vi "Update Form.vi"(7 "Name":string, 8 "error in (no error)":errorcluster, 10 "Table":refnum<class "Basic Table.lvclass">, 11 "Form Server Wrapper in":refnum<class "Form Server Wrapper.lvclass">) -> (0 "error out":errorcluster, 3 "Form Server Wrapper out":refnum<class "Form Server Wrapper.lvclass">)   [LabVIEW 2020, in "Form Server.lvlib" / "Form Server Wrapper.lvclass"]
uses:
  Form Server Wrapper.lvclass
  Database OOP/Table Libraries/Basic Table/Basic Table Class/Basic Table.lvclass
  Form Server Wrapper.lvclass/Form Server Wrapper.ctl
  Form Server Messages Messages/Update Form Msg/Update Form Msg.lvclass/Update Form Msg.ctl
  <vilib>/ActorFramework/Message Enqueuer/Message Enqueuer.lvclass/Message Enqueuer.ctl
  <vilib>/ActorFramework/Message Enqueuer/Enqueue.vi
  Form Server Messages Messages/Update Form Msg/Update Form Msg.lvclass
  C:/Program Files (x86)/National Instruments/LabVIEW 2020/vi.lib/ActorFramework/Message/Message.lvclass
  <vilib>/ActorFramework/Message Priority Queue/Priority Enqueue.vi
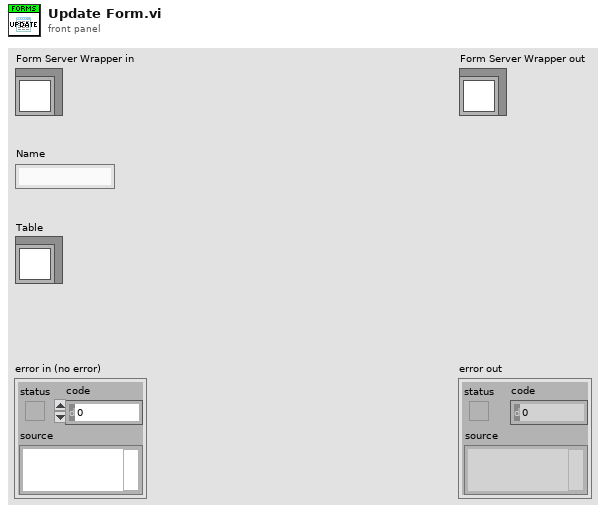
[diagram p1: front panel]
types:
  T1 = typedef "Form Server Interfaces.lvlib/Form ID.ctl" = cluster{"Name":string, "Panel type":string}
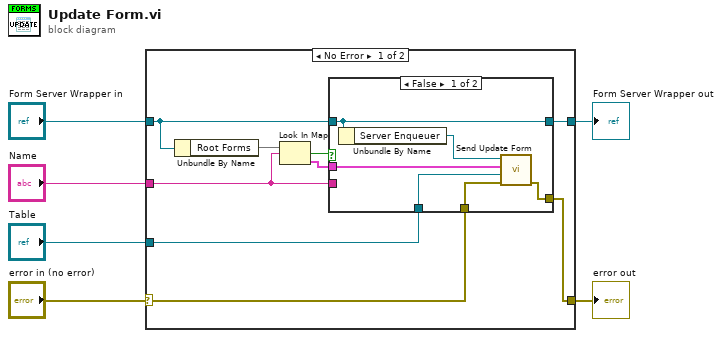
[diagram p0: block diagram]
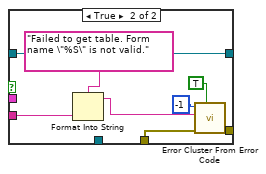
[diagram p2: hidden frame]
diagram:
  n1 = case shown="No Error" "error in (no error)" {
    selector: "error in (no error)" -> [w14 w31]
    tunnel: [w13 w31] -> w4
    tunnel: [w15 w30] -> w5
    tunnel: "Form Server Wrapper in" -> [w12 w30]
    tunnel: "Name" -> [w8 _]
    tunnel: "Table" -> [w7 _]
    frame No Error {
      n2 = Unbundle By Name(w12) -> ("Root Forms"=w11:map{string, T1})
      n3 = Look In Map(map=w11, key=w8) -> (key not found?=w10:bool, value=w9:T1)  [unwired: 1 in]
      n4 = case shown="False" w10 {
        tunnel: w9 -> [w19 _]
        tunnel: w12 -> [w21 w26]
        tunnel: [w21 w26] -> w15
        tunnel: w14 -> [w18 w29]
        tunnel: w8 -> [_ w24]
        tunnel: [w17 w22] -> w13
        tunnel: w7 -> [w16 _]
        frame False {
          n5 = Unbundle By Name(w21) -> ("Server Enqueuer"=w20:refnum<class "Message Enqueuer.lvclass">)
          n6 = call "Send Update Form.vi"("error in (no error)"=w18, "Table"=w16, "Form ID"=w19, "Message Enqueuer"=w20) -> ("error out"=w17:errorcluster)  [unwired: 6 in, 1 out]
        }
        frame True {
          n7 = Format Into String(format string="Failed to get table. Form name \"%S\" is not valid.", w24) -> (resulting string=w23:string)  [unwired: 2 in, 1 out]
          n8 = call <vilib>:"Error Cluster From Error Code.vi"("show call chain? (False)"=TRUE, "error in (no error)"=w29, "error message (\"\")"=w23, "error code (0)"=-1) -> ("error out"=w22:errorcluster)  [unwired: 5 in]
        }
      }
    }
    frame Error {
    }
  }
  "error out" <- w4
  "Form Server Wrapper out" <- w5
